vi "GetToolbarButtons.vi"(0 "reference in":refnum<class "ClassDiagramGraph.lvclass">, 2 "GraphButton":u32, 5 "error in (no error)":errorcluster) -> (14 "reference out":refnum<class "ClassDiagramGraph.lvclass">, 15 "ToolbarButtons":T2[](array[typedef]), 16 "Text":string, 17 "Type":T1, 19 "error out":errorcluster)   [LabVIEW 2020, in "ClassDiagramGraph.lvclass"]
uses:
  <resource>/Framework/Providers/Open_GDS/UML/ClassDiagramGraph_class/ClassDiagramGraph.lvclass
  <resource>/Framework/Providers/Open_GDS/UML/Graph_class/ToolbarButtonType.ctl
  <resource>/Framework/Providers/Open_GDS/UML/UMLEditor/UMLEditor tooltype.ctl
  <resource>/Framework/Providers/Open_GDS/UML/Graph_class/Graph.lvclass
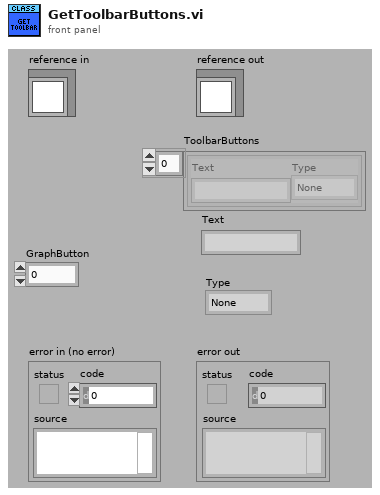
[diagram p1: front panel]
types:
  T1 = typedef "UMLEditor tooltype.ctl" = enum16{"None", "Node", "Edge"}
  T2 = typedef "Graph.lvclass/ToolbarButtonType.ctl" = cluster{"Text":string, "Type":T1}
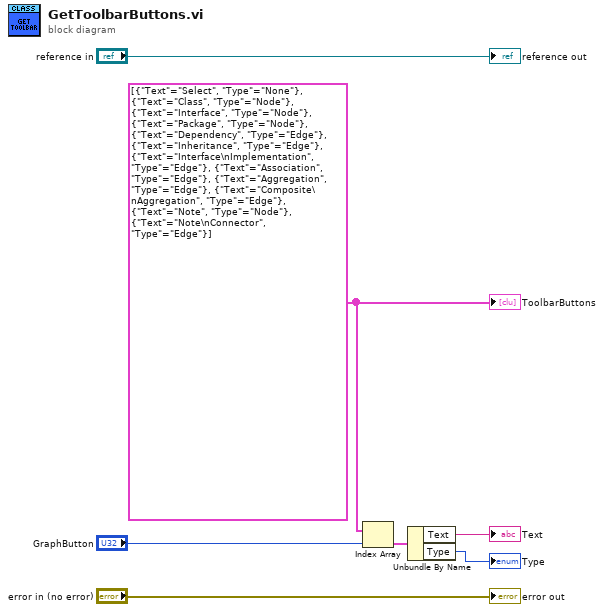
[diagram p0: block diagram]
diagram:
  w5 = T2[] [{"Text"="Select", "Type"=enum."None"}, {"Text"="Class", "Type"=enum."Node"}, {"Text"="Interface", "Type"=enum."Node"}, {"Text"="Package", "Type"=enum."Node"}, {"Text"="Dependency", "Type"=enum."Edge"}, {"Text"="Inheritance", "Type"=enum."Edge"}, {"Text"="Interface\nImplementation", "Type"=enum."Edge"}, {"Text"="Association", "Type"=enum."Edge"}, {"Text"="Aggregation", "Type"=enum."Edge"}, {"Text"="Composite\nAggregation", "Type"=enum."Edge"}, {"Text"="Note", "Type"=enum."Node"}, {"Text"="Note\nConnector", "Type"=enum."Edge"}] ("ToolbarButtons")
  n1 = Index Array(array=w5, index="GraphButton") -> (element=w3:T2)
  n2 = Unbundle By Name(w3) -> ("Text"=→"Text":string, "Type"=→"Type":T1)
  "error out" <- "error in (no error)"
  "reference out" <- "reference in"
  "ToolbarButtons" <- w5
